vi "Image to String.vi"(8 "error in (no error)":errorcluster, 10 "Image":T1, 11 "CameraDevRef":T2={"Camera Address"="192.168.0.90", "CameraStatus"={"status"=FALSE, "code"=0, "source"=""}}) -> (0 "error out":errorcluster, 2 "Image Data String":string, 3 "CameraDevRef Out":T2)   [LabVIEW 2015]
uses:
  <vilib>/Rock Robotics/WPI/Camera/WPI_CameraDevRef.ctl
  <vilib>/vision/Image Controls.llb/IMAQ Image.ctl
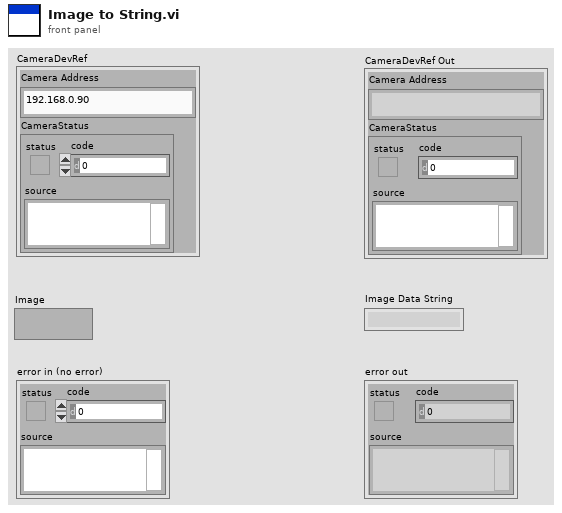
[diagram p1: front panel]
types:
  T1 = typedef "IMAQ Image.ctl" = refnum<image>
  T2 = typedef "WPI_CameraDevRef.ctl" = cluster{"Camera Address":string, "CameraStatus":errorcluster}
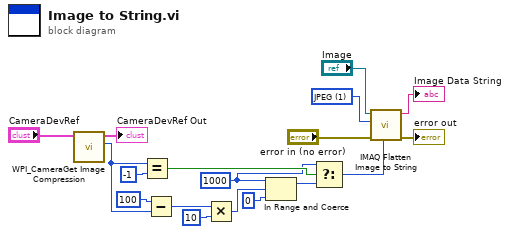
[diagram p0: block diagram]
diagram:
  w3 = 1000
  w18 = 1 items=["None", "JPEG", "PACKED BINARY"] ("Compression (None)")
  n1 = call <vilib>:"WPI_CameraGet Image Compression.vi"("CameraDevRef"="CameraDevRef") -> ("Compression"=w5:i32, "CameraDevRef Out"=→"CameraDevRef Out":T2)  [unwired: 8 in, 1 out]
  n2 = Equal?(x=w5, y=-1) -> (x = y?=w4:bool)
  n3 = Subtract(x=100, y=w5) -> (x-y=w14:i32)
  n4 = Multiply(x=w14, y=10) -> (x*y=w16:i32)
  n5 = In Range and Coerce(upper limit=w3, x=w16, lower limit=0) -> (coerced(x)=w2:i32)  [unwired: 1 out]
  n6 = Select(t=w3, s=w4, f=w2) -> (s? t:f=w1:i32)
  n7 = call "IMAQ Flatten Image to String"("Quality (750)"=w1, "error in (no error)"="error in (no error)", "Compression (None)"=w18, "Image"="Image") -> ("error out"=→"error out":errorcluster, "Data String"=→"Image Data String":string)  [unwired: 6 in]
